vi "GET_Travel_(offline).vi"(0 "Loaded.X in":dbl[](array[numeric]), 5 "Loaded.Y in":dbl[](array[numeric]), 7 "Loaded.Speed in":dbl[](array[numeric]), 9 "Speed threshold":dbl, 11 "Error In":errorcluster) -> (4 "Run length, m":dbl, 8 "Loaded.Speed out":dbl[](array[numeric]), 15 "Error Out":errorcluster)   [LabVIEW 2018, in "Tracker.lvlib"]
uses:
  Tracker.lvlib
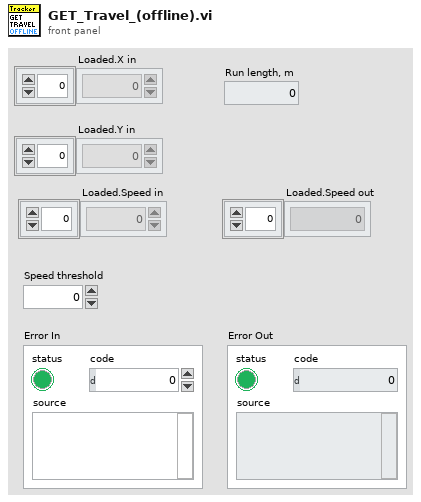
[diagram p1: front panel]
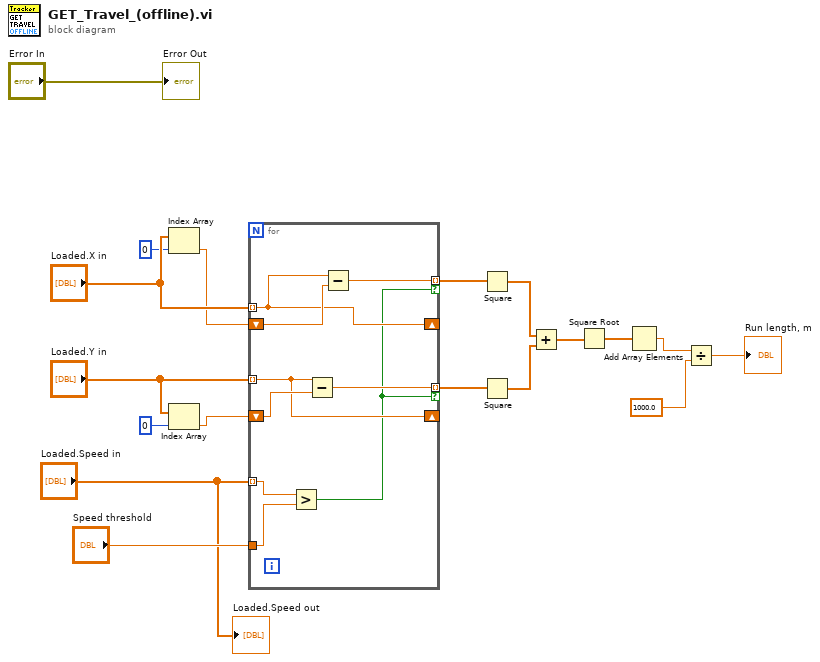
[diagram p0: block diagram]
diagram:
  n1 = Index Array(array="Loaded.X in", index=0) -> (element=w15:dbl)
  n2 = Index Array(array="Loaded.Y in", index=0) -> (element=w12:dbl)
  n3 = for {
    tunnel: "Loaded.X in" -> [w25] mode=indexing
    shift-right: [w25] -> _
    shift-left: w15 -> [w27]
    tunnel: [w26] -> w9 mode=indexing if=w19
    tunnel: "Loaded.Y in" -> [w22] mode=indexing
    shift-right: [w22] -> _
    shift-left: w12 -> [w24]
    tunnel: [w23] -> w8 mode=indexing if=w19
    tunnel: "Loaded.Speed in" -> [w21] mode=indexing
    tunnel: "Speed threshold" -> [w20]
    n4 = Greater?(x=w21, y=w20) -> (0:w19:bool)
    n5 = Subtract(x=w22, y=w24) -> (x-y=w23:dbl)
    n6 = Subtract(x=w25, y=w27) -> (x-y=w26:dbl)
  }
  n7 = Square(x=w9) -> (x^2=w7:dbl[])
  n8 = Square(x=w8) -> (x^2=w6:dbl[])
  n9 = Add(x=w7, y=w6) -> (x+y=w5:dbl[])
  n10 = Square Root(x=w5) -> (sqrt(x)=w4:dbl[])
  n11 = Add Array Elements(numeric array=w4) -> (sum=w3:dbl)
  n12 = Divide(x=w3, y=1000.0) -> (x/y=→"Run length, m":dbl)
  "Error Out" <- "Error In"
  "Loaded.Speed out" <- "Loaded.Speed in"
